vi "ParseVectorFile.NewFileSynchronous.vi"(6 "timeout in ms (-1)":i32=-1, 8 "error in (no error)":errorcluster, 10 "Path":path, 11 "ParseVectorFile":refnum<class "ParseVectorFile.lvclass">) -> (0 "error out":errorcluster, 2 "ParsedData":T1, 3 "ParseVectorFile out":refnum<class "ParseVectorFile.lvclass">)   [LabVIEW 2019, in "ParseVectorFile.lvclass"]
doc: "---------------------------------------------------------------\nJKI State Machine Objects™\nhttp://jki.net/state-machine-objects/\nCopyright (C) 2005-2015, JKI <info@jki.net>\nALL RIGHTS RESERVEDJKI State Machine Objects (SMO) 1.0.0.4\nJKI - JKI\nCopyright (c) 2015, JKI"
uses:
  ParseVectorFile.lvclass
  C:/Program Files (x86)/National Instruments/LabVIEW 2019/vi.lib/JKI/JKI SMO/SMO/SMO.lvclass
  Typedefs/PublicEvents--ParseVectorFile.ParsedData.ctl
  Image/SVGImage.lvclass
  ParseVectorFile.lvclass/ParseVectorFile.ctl
  Typedefs/PrivateEvents--ParseVectorFile.New File Synchronous.ctl
  ParsePaths/Path.lvclass
  Rectangle/Rectangle.lvclass
  <vilib>/JKI/JKI SMO/SMO/SMO.lvclass
  Dot/Dot.lvclass
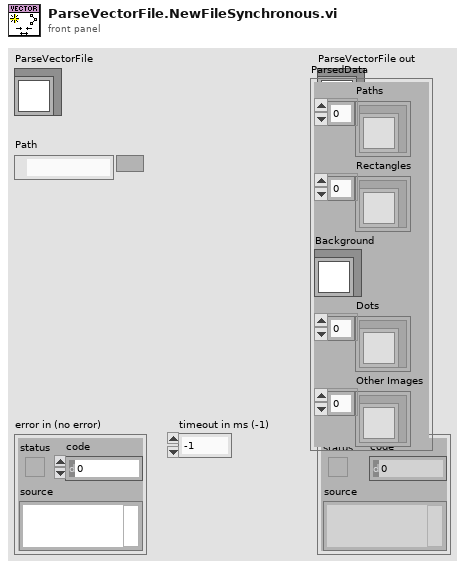
[diagram p1: front panel]
types:
  T1 = typedef "ParseVectorFile.lvclass/PublicEvents--ParseVectorFile.ParsedData.ctl" = cluster{"Paths":refnum<class "Path.lvclass">[], "Rectangles":refnum<class "Rectangle.lvclass">[], "Background":refnum<class "SVGImage.lvclass">, "Dots":refnum<class "Dot.lvclass">[], "Other Images":refnum<class "SVGImage.lvclass">[]}
  T2 = typedef "ParseVectorFile.lvclass/PrivateEvents--ParseVectorFile.New File Synchronous.ctl" = cluster{"Path":path, "Parsed Data":refnum<notifier>}
  T3 = typedef "SMO.lvclass/SMOState --Enum.ctl" = enum16{"unknown", "Created", "Started", "Stopped"}
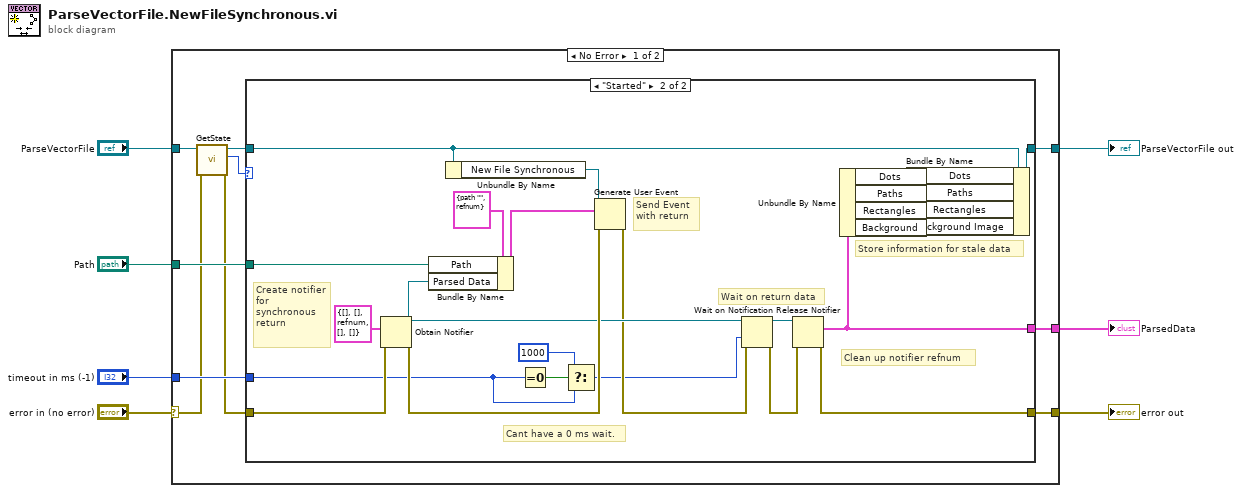
[diagram p0: block diagram]
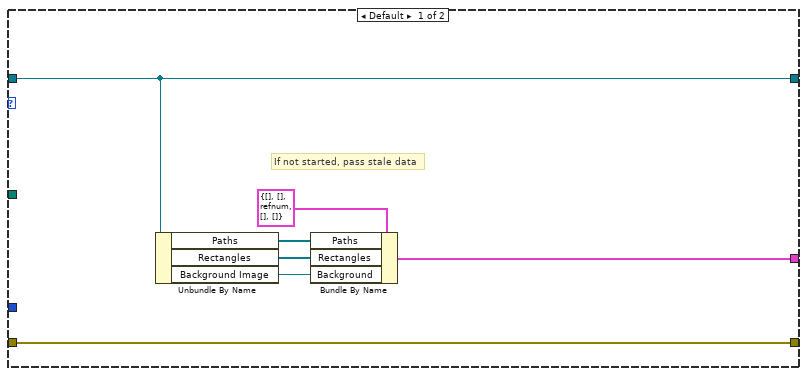
[diagram p2: hidden frame]
diagram:
  n1 = case shown="No Error" "error in (no error)" {
    selector: "error in (no error)" -> [w9 w49]
    tunnel: [w17 w49] -> w6
    tunnel: [w16 w48] -> w7
    tunnel: "ParseVectorFile" -> [w14 w48]
    tunnel: "Path" -> [w12 _]
    tunnel: "timeout in ms (-1)" -> [w11 _]
    tunnel: [w10 _] -> w2
    frame No Error {
      n2 = call <vilib>:"GetState.vi"("error in (no error)"=w9, "SMO"=w14) -> ("error out"=w8:errorcluster, "SMO State"=w13:T3, "SMO out"=w15:refnum<class "ParseVectorFile.lvclass">)  [unwired: 7 in]
      n3 = case shown="\"Started\"" w13 {
        tunnel: w8 -> [w24 w42]
        tunnel: [w24 w32] -> w17
        tunnel: w15 -> [w23 w29]
        tunnel: [w23 w30] -> w16
        tunnel: w12 -> [_ w46]
        tunnel: w11 -> [_ w36]
        tunnel: [w18 w31] -> w10
        frame Default {
          # "If not started, pass stale data"
          n4 = Unbundle By Name(w23) -> ("Paths"=w21:refnum<class "Path.lvclass">[], "Rectangles"=w20:refnum<class "Rectangle.lvclass">[], "Background Image"=w19:refnum<class "SVGImage.lvclass">)
          n5 = Bundle By Name(cluster=T1 {"Paths"=[], "Rectangles"=[], "Background"=refnum, "Dots"=[], "Other Images"=[]} ("ParsedData"), "Paths"=w21, "Rectangles"=w20, "Background"=w19) -> (w18:T1)
        }
        frame "Started" {
          # "Store information for stale data"
          # "Clean up notifier refnum"
          # "Wait on return data"
          # "Send Event with return"
          # "Create notifier for synchronous return"
          # "Cant have a 0 ms wait."
          n6 = Obtain Notifier(notification data type=T1 {"Paths"=[], "Rectangles"=[], "Background"=refnum, "Dots"=[], "Other Images"=[]} ("ParsedData"), error in (no error)=w42) -> (notifier out=w41:refnum<notifier>, error out=w43:errorcluster)  [unwired: 2 in, 1 out]
          n7 = Bundle By Name(cluster=T2 {"Path"=path "", "Parsed Data"=refnum} ("New File Synchronous"), "Path"=w46, "Parsed Data"=w41) -> (w40:T2)
          n8 = Unbundle By Name(w29) -> ("New File Synchronous"=w45:refnum<user-event>)
          n9 = Equal To 0?(x=w36) -> (x = 0?=w38:bool)
          n10 = Select(t=1000, s=w38, f=w36) -> (s? t:f=w35:i32)
          n11 = Generate User Event(user event=w45, event data cluster=w40, error in=w43) -> (error out=w39:errorcluster)  [unwired: 1 in, 1 out]
          n12 = Wait on Notification(notifier=w41, timeout in ms (-1)=w35, error in (no error)=w39) -> (notifier out=w34:refnum<notifier>, error out=w33:errorcluster)  [unwired: 1 in, 2 out]
          n13 = Release Notifier(notifier=w34, error in (no error)=w33) -> (last notification=w31:T1, error out=w32:errorcluster)  [unwired: 1 in, 1 out]
          n14 = Unbundle By Name(w31) -> ("Dots"=w25:refnum<class "Dot.lvclass">[], "Paths"=w26:refnum<class "Path.lvclass">[], "Rectangles"=w27:refnum<class "Rectangle.lvclass">[], "Background"=w28:refnum<class "SVGImage.lvclass">)
          n15 = Bundle By Name(cluster=w29, "Dots"=w25, "Paths"=w26, "Rectangles"=w27, "Background Image"=w28) -> (w30:refnum<class "ParseVectorFile.lvclass">)
        }
      }
    }
    frame Error {
    }
  }
  "error out" <- w6
  "ParseVectorFile out" <- w7
  "ParsedData" <- w2
